vi "iWorx - Gas Pressure_X.vi"() -> ()   [LabVIEW 2012]
uses:
  <vilib>/DAQmx/create/channels.llb/DAQmx Create Channel (AI-Voltage-Basic).vi
  <vilib>/DAQmx/read.llb/DAQmx Read (Analog 1D Wfm NChan 1Samp).vi
panel:
  out "Offset":dbl=10.0
  out "Slope":dbl=50.0
  in  "Set SP2":bool
  in  "Set SP1":bool
  in  "Calibration Data":T1={"SP1 Voltage"=5.0, "SP2 Voltage"=0.0, "SP1 Value"=260.0, "SP2 Value"=10.0} {"SP2 Voltage" format="%#_g V"; "SP1 Voltage" format="%#_g V"}
  in  "Set Up":bool
  in  "Channel":u16(ring) items=["Channel 1", "Channel 2"]
  in  "Pause Button":bool
  in  "Snapshot":bool
  out "Processed Signal":dbl(knob) caption="Pressure" scale=0.0..1000.0
  in  "stop":bool
  out "Waveform Chart":waveform(dbl)(graph)
  in  "Sample Timing":u16(ring)=200 items=["20Hz"=50, "5 Hz"=200, "2 Hz"=500, "1 Hz"=1000, ".5 Hz"=2000, ".2 Hz"=5000]
  in  "Clear Chart":bool
  in  "Open Log":bool
  in  "Autoscale Y":bool
  out "Raw Signal":dbl(knob) scale=-5.0..5.0
  # "iWorx - Gas Pressure - Data Logger"
  # "Sensor Input"
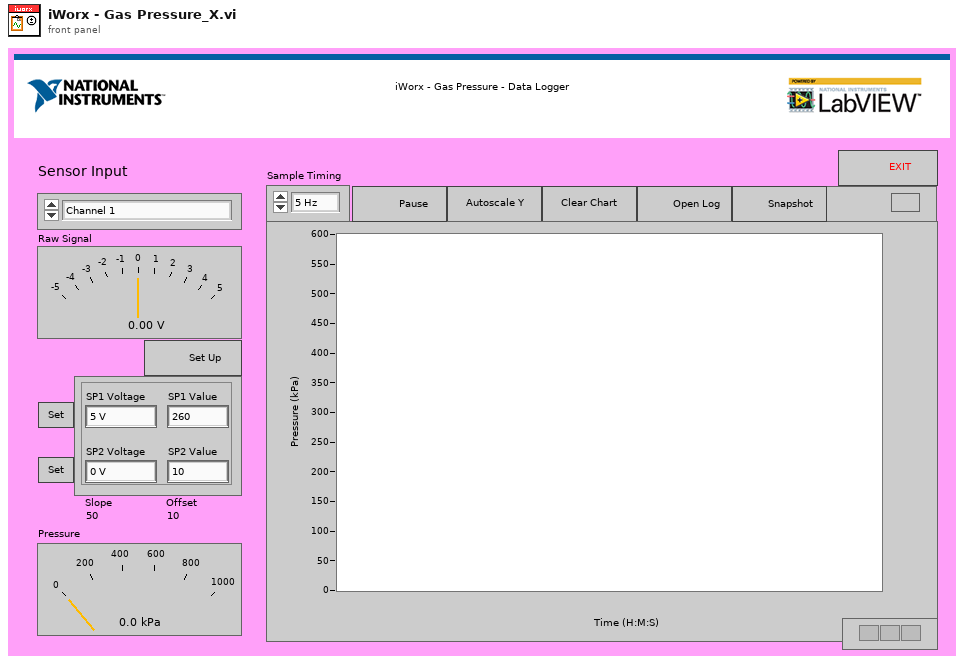
[diagram p1: front panel]
types:
  T1 = cluster{"SP1 Voltage":dbl, "SP2 Voltage":dbl, "SP1 Value":dbl, "SP2 Value":dbl}
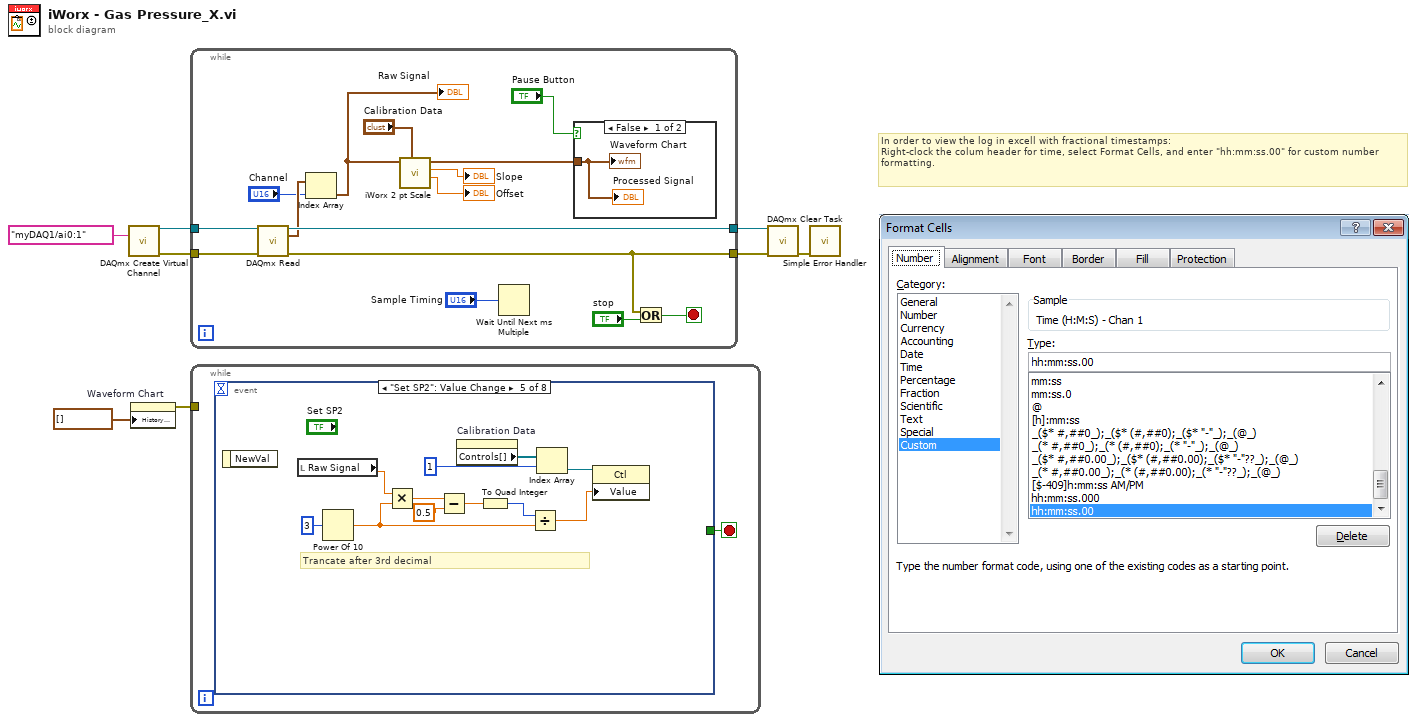
[diagram p0: block diagram]
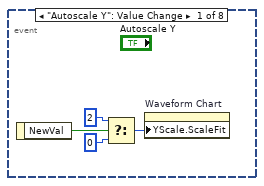
[diagram p2: hidden frame]
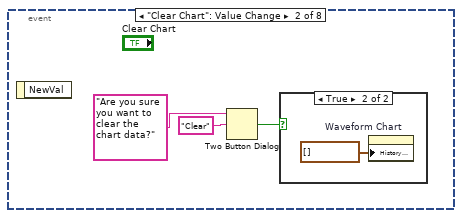
[diagram p3: hidden frame]
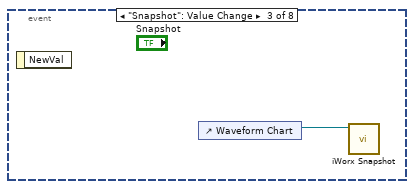
[diagram p5: hidden frame]
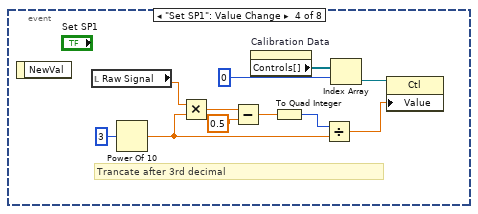
[diagram p6: hidden frame]
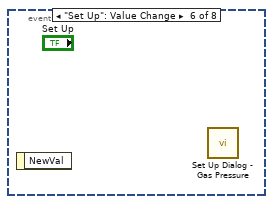
[diagram p7: hidden frame]
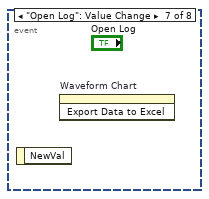
[diagram p8: hidden frame]
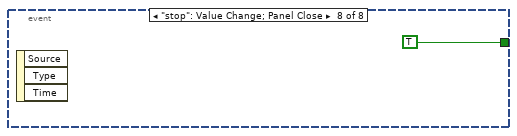
[diagram p9: hidden frame]
diagram:
  # "In order to view the log in excell with fractional timestamps: \nRight-clock the colum header for time, select Format Cells, and enter \"hh:mm:ss.00\" for custom number formatting."
  n1 = call-poly <vilib>:"DAQmx Create Virtual Channel.vi"("physical channels"=tag "myDAQ1/ai0:1") -> ("task out"=w5:refnum<k21>, "error out"=w4:errorcluster)  [unwired: 13 in]
  n2 = property on="Waveform Chart" class="WFChart (strict)"("History Data"=waveform(dbl)[] []) -> (error out=w3:errorcluster)  [unwired: 2 in, 1 out]
  n3 = while {
    tunnel: w5 -> [w21]
    tunnel: [w20] -> w8
    tunnel: w4 -> [w19]
    tunnel: [w17] -> w7
    stop <- w18 stop-if-true
    n4 = call-poly <vilib>:"DAQmx Read.vi"("task/channels in"=w21, "error in"=w19) -> ("task out"=w20:refnum<k21>, "data"=w15:waveform(dbl)[], "error out"=w17:errorcluster)  [unwired: 11 in]
    n5 = Index Array(array=w15, index="Channel") -> (element=w13:waveform(dbl))
    "Raw Signal" <- w13
    n6 = call "iWorx 2 pt Scale.vi"("Set Points"="Calibration Data", "Raw Waveform"=w13) -> ("Offset"=→"Offset":dbl, "Slope"=→"Slope":dbl, "Scaled Value"=w14:waveform(dbl))  [unwired: 7 in]
    n7 = Wait Until Next ms Multiple(millisecond multiple="Sample Timing") -> ()  [unwired: 1 out]
    n8 = case shown="False" "Pause Button" {
      tunnel: w14 -> [w24 _]
      frame False {
        "Waveform Chart" <- w24
        "Processed Signal" <- w24
      }
      frame True {
      }
    }
    n9 = Or(x=w17, y="stop") -> (x .or. y?=w18:bool)
  }
  n10 = while {
    tunnel: w3 -> [_]
    stop <- w25 stop-if-true
    n11 = event shown="[4] \"Set SP2\": Value Change" {
      selector: _ -> [_ _ _ _ _ _ _ _]
      dyn-events: _ -> [_ _ _ _ _ _ _ _]
      timeout: _ -> [_ _ _ _ _ _ _ _]
      tunnel: [_ _ _ _ _ _ _ TRUE] -> w25
      event "Autoscale Y": Value Change {
        n12 = event-data() -> ("NewVal"=w27:bool)  [unwired: 1 in]
        n13 = Select(t=u8 2 ("Y Scale.Scale Fit"), s=w27, f=u8 0 ("Y Scale.Scale Fit")) -> (s? t:f=w26:u8)
        n14 = property on="Waveform Chart" class="WFChart (strict)"("YScale.ScaleFit"=w26) -> ()  [unwired: 2 in, 2 out]
      }
      event "Clear Chart": Value Change {
        n15 = event-data() -> ()  [unwired: 1 in, 1 out]
        n16 = Two Button Dialog(message="Are you sure you want to clear the chart data?", 2:"Clear" ("T button name (\"OK\")")) -> (T button?=w31:bool)  [unwired: 1 in]
        n17 = case shown="True" w31 {
          frame False {
          }
          frame True {
            n18 = property on="Waveform Chart" class="WFChart (strict)"("History Data"=waveform(dbl)[] []) -> ()  [unwired: 2 in, 2 out]
          }
        }
      }
      event "Snapshot": Value Change {
        n19 = event-data() -> ()  [unwired: 1 in, 1 out]
        n20 = control-ref of="Waveform Chart"() -> (w34:refnum<vi>)
        n21 = call "iWorx Snapshot.vi"("WaveformChart in"=w34) -> ()  [unwired: 10 in, 1 out]
      }
      event "Set SP1": Value Change {
        # "Trancate after 3rd decimal"
        n22 = event-data() -> ()  [unwired: 1 in, 1 out]
        n23 = local read "Raw Signal"() -> (w45:dbl)
        n24 = Power Of 10(x=3) -> (10^x=w38:dbl)
        n25 = Multiply(x=w45, y=w38) -> (x*y=w40:dbl)
        n26 = Subtract(x=w40, y=0.5) -> (x-y=w41:dbl)
        n27 = property on="Calibration Data" class="Clust (strict)"() -> ("Controls[]"=w35:refnum<vi>[])  [unwired: 2 in, 2 out]
        n28 = To Quad Integer(1:w41) -> (0:w39:i64)
        n29 = Divide(x=w39, y=w38) -> (x/y=w43:dbl)
        n30 = Index Array(array=w35, index=0) -> (element=w36:refnum<vi>)
        n31 = property class="Ctl"(reference=w36, "Value"=w43) -> ()  [unwired: 1 in, 2 out]
      }
      event "Set SP2": Value Change {
        # "Trancate after 3rd decimal"
        n32 = event-data() -> ()  [unwired: 1 in, 1 out]
        n33 = local read "Raw Signal"() -> (w56:dbl)
        n34 = Power Of 10(x=3) -> (10^x=w49:dbl)
        n35 = Multiply(x=w56, y=w49) -> (x*y=w51:dbl)
        n36 = Subtract(x=w51, y=0.5) -> (x-y=w52:dbl)
        n37 = property on="Calibration Data" class="Clust (strict)"() -> ("Controls[]"=w46:refnum<vi>[])  [unwired: 2 in, 2 out]
        n38 = To Quad Integer(1:w52) -> (0:w50:i64)
        n39 = Divide(x=w50, y=w49) -> (x/y=w54:dbl)
        n40 = Index Array(array=w46, index=1) -> (element=w47:refnum<vi>)
        n41 = property class="Ctl"(reference=w47, "Value"=w54) -> ()  [unwired: 1 in, 2 out]
      }
      event "Set Up": Value Change {
        n42 = event-data() -> ()  [unwired: 1 in, 1 out]
        n43 = call "Set Up Dialog - Gas Pressure.vi"() -> ()  [unwired: 12 in]
      }
      event "Open Log": Value Change {
        n44 = event-data() -> ()  [unwired: 1 in, 1 out]
        n45 = invoke on="Waveform Chart" class="WFChart (strict)" method="Export Data to Excel"() -> ()  [unwired: 3 in, 3 out]
      }
      event "stop": Value Change; Panel Close {
        n46 = event-data() -> ()  [unwired: 1 in, 3 out]
      }
    }
  }
  n47 = call <vilib>:"DAQmx Clear Task.vi"("task in"=w8, "error in"=w7) -> ("error out"=w2:errorcluster)  [unwired: 13 in]
  n48 = call <vilib>:"Simple Error Handler.vi"("error in (no error)"=w2) -> ()  [unwired: 4 in, 5 out]
